vi "FTW-Ether-Construct.vi"(5 "FTW Ether Configuration":string="{\n  \"ApplicationName\": \"Featherweight Application\",\n  \"ApplicationVersion\": \"0.1.0-1\",\n  \"LoggerAddress\": \"tcp://127.0.0.1:*\",\n  \"LoggerName\": \"Log\",\n  \"LoggerDirectory\": \"[UserAppData]\\\\Featherweight\\\\Logs\",\n  \"LoggerDiskThrashDelay\": 200\n}", 11 "error in":errorcluster) -> (15 "error out":errorcluster)   [LabVIEW 2012, in "FTW-Actor.lvlib" / "FTW-Ether.lvclass"]
uses:
  FTW-Ether.lvclass
  Core/src/Reflection/FTW-Reflection-Type.vi
  Core/src/JSON/FTW-JSON-Core-LibraryFilepath.vi
  Core/src/JSON/FTW-JSON-Core-GetFlattenedValue.vi
  Core/src/JSON/FTW-JSON-Core-LibraryError.vi
  FTW-Ether-Instance.vi
  Core/utils/CodeGen/JSON Deserialize/FTW-JSON-Deserialize.xnode
  EventLogger/FTW-Logger.lvclass
panel:
  # "Inputs"
  # "Outputs"
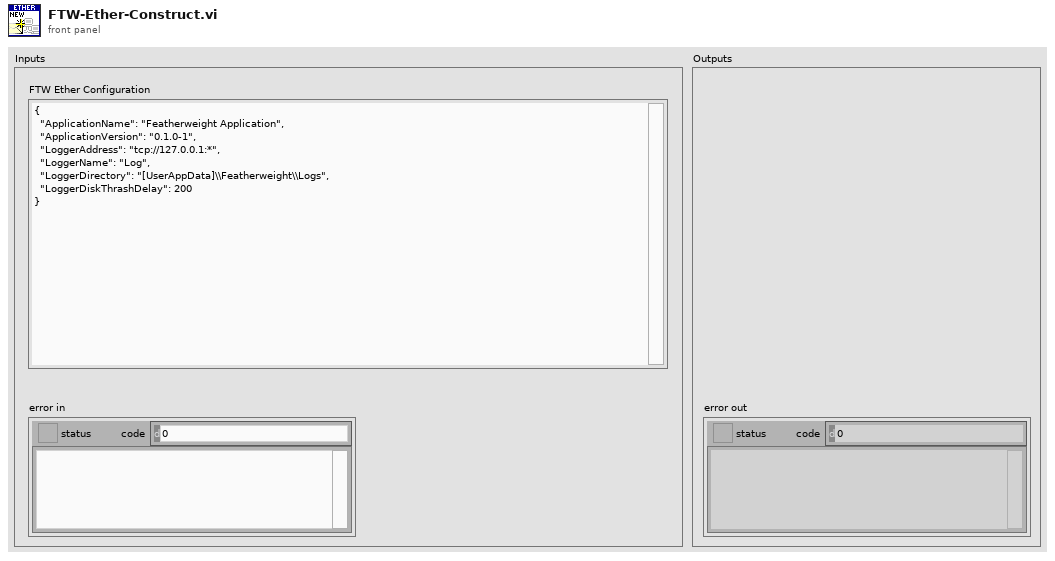
[diagram p1: front panel]
types:
  T1 = cluster{"ApplicationName":string, "ApplicationVersion":string, "LoggerAddress":string, "LoggerName":string, "LoggerDirectory":path, "LoggerDiskThrashDelay":u32}
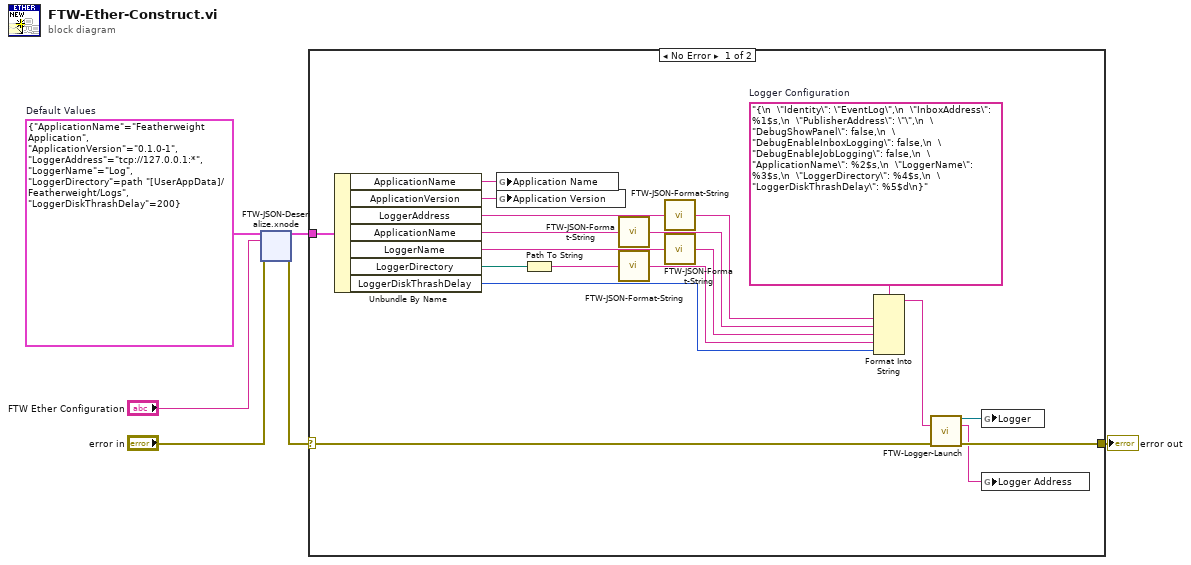
[diagram p0: block diagram]
diagram:
  w1 = T1 {"ApplicationName"="Featherweight Application", "ApplicationVersion"="0.1.0-1", "LoggerAddress"="tcp://127.0.0.1:*", "LoggerName"="Log", "LoggerDirectory"=path "[UserAppData]/Featherweight/Logs", "LoggerDiskThrashDelay"=200}  # Default Values
  n1 = xnode "FTW-JSON-Deserialize.xnode"("Type and Defaults"=w1, "JSON String"="FTW Ether Configuration", "error in"="error in") -> ("Values"=w2:T1, "error out"=w3:errorcluster)
  n2 = case shown="No Error" w3 {
    selector: w3 -> [w7 w26]
    tunnel: [w25 w26] -> w6
    tunnel: w2 -> [w18 _]
    frame No Error {
      w22 = "{\n  \"Identity\": \"EventLog\",\n  \"InboxAddress\": %1$s,\n  \"PublisherAddress\": \"\",\n  \"DebugShowPanel\": false,\n  \"DebugEnableInboxLogging\": false,\n  \"DebugEnableJobLogging\": false,\n  \"ApplicationName\": %2$s,\n  \"LoggerName\": %3$s,\n  \"LoggerDirectory\": %4$s,\n  \"LoggerDiskThrashDelay\": %5$d\n}"  # Logger Configuration
      n3 = Unbundle By Name(w18) -> ("ApplicationName"=w24:string, "ApplicationVersion"=w23:string, "LoggerAddress"=w10:string, "ApplicationName"=w12:string, "LoggerName"=w14:string, "LoggerDirectory"=w16:path, "LoggerDiskThrashDelay"=w17:u32)
      n4 = global write "FTW-Ether-Instance.vi" "Application Name"(w24) -> ()
      n5 = global write "FTW-Ether-Instance.vi" "Application Version"(w23) -> ()
      n6 = Path To String(path=w16) -> (string=w8:string)
      n7 = call "FTW-JSON-Format-String.vi"("LabVIEW String"=w12) -> ("JSON String"=w11:string)
      n8 = call "FTW-JSON-Format-String.vi"("LabVIEW String"=w8) -> ("JSON String"=w15:string)
      n9 = call "FTW-JSON-Format-String.vi"("LabVIEW String"=w10) -> ("JSON String"=w9:string)
      n10 = call "FTW-JSON-Format-String.vi"("LabVIEW String"=w14) -> ("JSON String"=w13:string)
      n11 = Format Into String(format string=w22, w9, w11, w13, w15, w17) -> (resulting string=w21:string)  [unwired: 2 in, 1 out]
      n12 = call "FTW-Logger-Launch.vi"("FTW Logger Configuration"=w21, "error in"=w7) -> ("FTW Logger Connector"=w20:refnum<class "FTW-Logger.lvclass">, "Logger Address"=w19:string, "error out"=w25:errorcluster)  [unwired: 11 in]
      n13 = global write "FTW-Ether-Instance.vi" "Logger"(w20) -> ()
      n14 = global write "FTW-Ether-Instance.vi" "Logger Address"(w19) -> ()
    }
    frame Error {
    }
  }
  "error out" <- w6
